vi "Write Font.vi"(8 "error in (no error)":errorcluster, 10 "Font Class.lvclass":refnum<class "Font Class.lvclass">, 11 "PDF Report Class in":refnum<class "PDF Report Class.lvclass">) -> (0 "error out":errorcluster, 3 "PDF Report Class out":refnum<class "PDF Report Class.lvclass">)   [LabVIEW 2019, in "Exaprom PDF.lvlib" / "PDF Report Class.lvclass"]
uses:
  PDF Report Class.lvclass
  Fonts Class/Font Class.lvclass
  PDF Report Class.lvclass/PDF Report Class.ctl
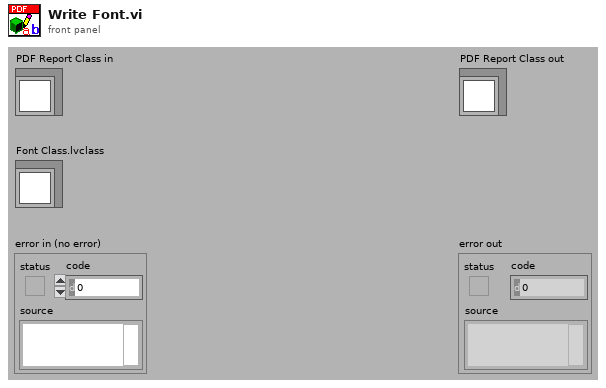
[diagram p1: front panel]
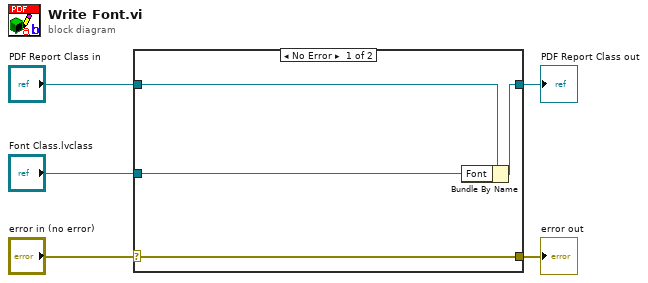
[diagram p0: block diagram]
diagram:
  n1 = case shown="No Error" "error in (no error)" {
    selector: "error in (no error)" -> [w9 w10]
    tunnel: [w9 w10] -> w4
    tunnel: [w7 w11] -> w2
    tunnel: "PDF Report Class in" -> [w8 w11]
    tunnel: "Font Class.lvclass" -> [w6 _]
    frame No Error {
      n2 = Bundle By Name(cluster=w8, "Font"=w6) -> (w7:refnum<class "PDF Report Class.lvclass">)
    }
    frame Error {
    }
  }
  "error out" <- w4
  "PDF Report Class out" <- w2
